vi "Webcam_Close.vi"(8 "error in (no error)":errorcluster) -> (0 "error out":errorcluster)   [LabVIEW 2014, in "QwaveSys RPi Training Library.lvlib"]
uses:
  <vilib>/Q-Wave Systems/QwaveSys RPi Package 2.0/Addons/QwaveSys RPi Training Library.lvlib
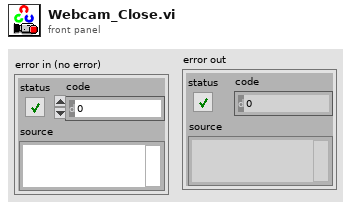
[diagram p1: front panel]
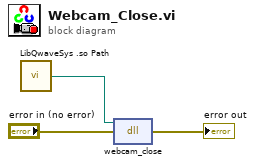
[diagram p0: block diagram]
diagram:
  n1 = call <vilib>:"LibQwaveSys .so Path.vi"() -> ("Lib QwaveSys .so Path"=w1:path)  [unwired: 5 in]
  n2 = dll-call lib="libqwavesys.so" fn="webcam_close"(path in=w1, error in="error in (no error)") -> (error out=→"error out":errorcluster)  [unwired: 2 in, 1 out]
